vi "test Write and Read Single Array.vi"(8 "error in (no error)":errorcluster, 11 "TestCase in":refnum<class "Read Value Tests.lvclass">) -> (0 "error out":errorcluster, 3 "TestCase out":refnum<class "Read Value Tests.lvclass">)   [LabVIEW 2017, in "Read Value Tests.lvclass"]
uses:
  Read Value Tests.lvclass
  <vilib>/NI/Memory Manager/Classes/Pointer/Pointer.lvclass/Pointer.ctl
  <vilib>/NI/Memory Manager/Classes/Pointer/Protected/Parameter Checking/Check Null Pointer.vi
  <vilib>/NI/Memory Manager/Classes/Pointer/Private/Deallocate.vi
  <vilib>/NI/Memory Manager/Classes/Pointer/Protected/Errors.vi
  <vilib>/NI/Memory Manager/Classes/Pointer/Protected/Error VIs/Null Pointer.vi
  <vilib>/NI/Memory Manager/Classes/Pointer/API/Accessors/Get Address.vi
  <vilib>/NI/Memory Manager/Classes/Pointer/Protected/Get Internal.vi
  <vilib>/NI/Memory Manager/Classes/Pointer/Protected/Error VIs/Zone.vi
  <vilib>/NI/Memory Manager/Classes/Pointer/API/Accessors/Set Address.vi
  <vilib>/NI/Memory Manager/Classes/Pointer/API/Accessors/Set Size.vi
  <vilib>/NI/Memory Manager/Classes/Pointer/Private/Set Internal.vi
  <vilib>/NI/Memory Manager/Classes/Pointer/Protected/Error Building/Create Error.vi
  <vilib>/NI/Memory Manager/Constants/Constants.vi
  <vilib>/NI/Memory Manager/Constants/Library Name.vi
  <vilib>/NI/Memory Manager/Classes/Pointer/Protected/Error Building/Get Error Info.vi
  <vilib>/NI/Memory Manager/VIs/Write String into Source.vi
  <vilib>/NI/Memory Manager/VIs/Create Error Cluster.vi
  <vilib>/NI/Memory Manager/VIs/VIs for Poly/Create Error Cluster (256B).vi
  <vilib>/NI/Memory Manager/VIs/Set Error Status.vi
  <vilib>/NI/Memory Manager/VIs/Set Error Code.vi
  <vilib>/NI/Memory Manager/VIs/Set Error Source.vi
  Engine/Classes/Buffer/Buffer.lvclass
  C:/Program Files (x86)/National Instruments/LabVIEW 2017/vi.lib/NI/Memory Manager/Classes/Pointer/Pointer.lvclass
  Engine/Classes/Buffer/Read 1D SGL.vi
  <vilib>/addons/_JKI Toolkits/VI Tester/TestCase.llb/TestCase.lvclass
  <vilib>/NI/Memory Manager/Classes/Pointer/Pointer.lvclass
  C:/Program Files (x86)/National Instruments/LabVIEW 2017/vi.lib/addons/_JKI Toolkits/VI Tester/TestCase.llb/TestCase.lvclass
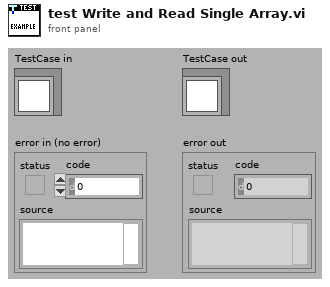
[diagram p1: front panel]
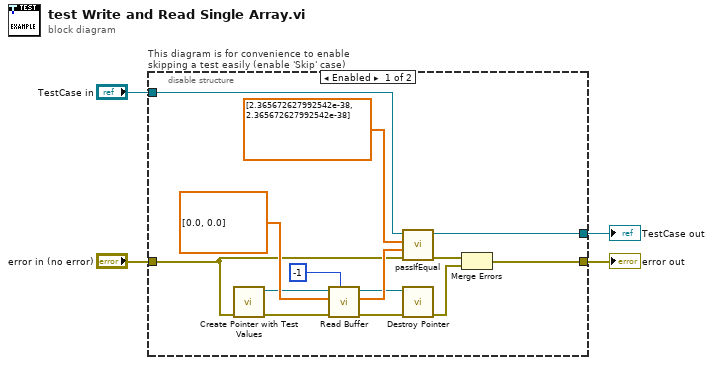
[diagram p0: block diagram]
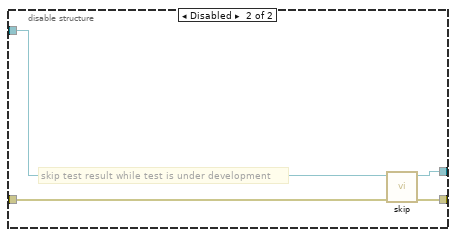
[diagram p2: hidden frame]
diagram:
  n1 = disable-structure "This diagram is for convenience to enable skipping a test easily (enable 'Skip' case)" shown="Enabled" {
    disable-tunnel: "TestCase in" -> [w11 w22]
    disable-tunnel: [w16 w20] -> w1
    disable-tunnel: [w15 w21] -> w3
    disable-tunnel: "error in (no error)" -> [w7 w19]
    frame Enabled {
      n2 = call "Create Pointer with Test Values.vi"("error in (no error)"=w7) -> ("error out"=w8:errorcluster, "Buffer out"=w9:refnum<class "Buffer.lvclass">)  [unwired: 9 in]
      n3 = call-poly "Read Buffer.vi"("count"=i64 -1, "error in (no error)"=w8, "buffer in"=sgl[] [0.0, 0.0], "Buffer in"=w9) -> ("error out"=w12:errorcluster, "buffer out"=w13:sgl[], "Buffer out"=w5:refnum<class "Buffer.lvclass">)  [unwired: 4 in, 1 out]
      n4 = call-dynamic "passIfEqual.vi"("error in (no error)"=w7, "y"=w13, "x"=sgl[] [2.3656726e-38, 2.3656726e-38] ("*(type *) &x"), "TestCase in"=w11) -> ("error out"=w17:errorcluster, "TestCase out"=w16:refnum<class "Read Value Tests.lvclass">)  [unwired: 6 in]
      n5 = call <vilib>:"Destroy Pointer.vi"("error in (no error)"=w12, "Pointer in"=w5) -> ("error out"=w6:errorcluster)  [unwired: 8 in, 1 out]
      n6 = Merge Errors(w17, w6) -> (w15:errorcluster)
    }
    frame Disabled {
      # "skip test result while test is under development"
      n7 = call <vilib>:"skip.vi"("error in (no error)"=w19, "TestCase in"=w22) -> ("error out"=w21:errorcluster, "TestCase out"=w20:refnum<class "Read Value Tests.lvclass">)  [unwired: 8 in]
    }
  }
  "error out" <- w3
  "TestCase out" <- w1
